vi "Get Movables.vi"(11 "Game Board in":refnum<class "Game Board.lvclass">) -> (2 "Movables out":refnum<class "Movable.lvclass">[](array[class]))   [LabVIEW 2021, in "Game Board.lvclass"]
doc: "MIT Licence\nCopyright (c) 2024 David Grollier"
uses:
  Game Board.lvclass
  Game Board Component/Movable/Movable.lvclass
  Game Board.lvclass/Game Board.ctl
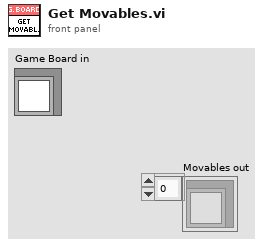
[diagram p1: front panel]
types:
  T1 = map{string, refnum<class "Game Board Component.lvclass">}
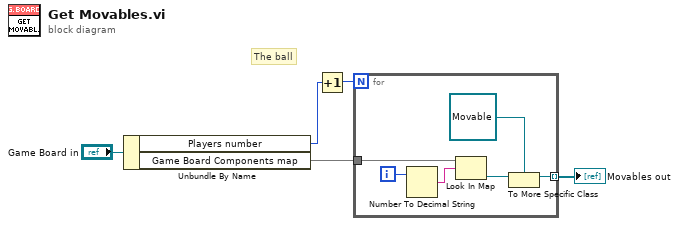
[diagram p0: block diagram]
diagram:
  # "The ball"
  n1 = Unbundle By Name("Game Board in") -> ("Players number"=w2:u8, "Game Board Components map"=w4:T1)
  n2 = Increment(x=w2) -> (x+1=w1:u8)
  n3 = for {
    N: w1 -> [_]
    tunnel: w4 -> [w11]
    tunnel: [w6] -> w3 mode=indexing
    i -> [w10]
    n4 = Number To Decimal String(number=w10) -> (decimal integer string=w9:string)  [unwired: 1 in]
    n5 = Look In Map(map=w11, key=w9) -> (value=w7:refnum<class "Game Board Component.lvclass">)  [unwired: 1 in, 1 out]
    n6 = To More Specific Class(target class=refnum<class "Movable.lvclass"> refnum ("Movable in"), reference=w7) -> (specific class reference=w6:refnum<class "Movable.lvclass">)  [unwired: 1 in, 1 out]
  }
  "Movables out" <- w3
